vi "VirtualChannelWhiteListProperties.vi"() -> (3 "virtual channel white list properties":string[](array[string]))   [LabVIEW 2017, in "DataExplorerSupport.lvlib"]
uses:
  <vilib>/addons/InsightCM/Utilities/DataExplorerSupport/DataExplorerSupport.lvlib
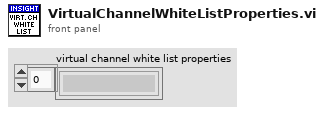
[diagram p1: front panel]
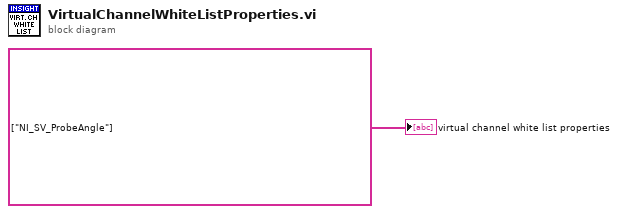
[diagram p0: block diagram]
diagram:
  "virtual channel white list properties" <- string[] ["NI_SV_ProbeAngle"] ("virtual channel white list properties")
